vi "Section 1.vi"() -> ()   [LabVIEW 2016]
panel:
  in  "Section Name 1":string
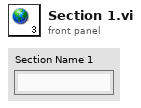
[diagram p1: front panel]
diagram:
